vi "Playback.vi"() -> ()   [LabVIEW 2018]
doc: "This VI reads records of data from the logging table in the LabVIEW.mdb database. \n\nAll the records from the table are retrieved at one time using the DB Tools Select Data VI. This data is in the format of a two dimensional array of variants. This array is indexed and each of the values are converted back to their original data types."
uses:
  database example subvis/Fetching - State.ctl
  <vilib>/addons/database/Connection.llb/Conn ObjectReference.ctl
  <vilib>/addons/database/Connection.llb/DB Tools Open Connec (Path).vi
  <vilib>/addons/database/_DB Variant To Data/Database Variant To Data.xnode
  <vilib>/addons/database/NI_Database_API.lvlib
panel:
  out "record number":i32
  in  "Previous Record":bool
  in  "Next Record":bool
  in  "Stop":bool
  out "min temperature value":dbl format="%#.6g"
  out "max temperature value":dbl format="%#.6g"
  out "min pressure value":dbl format="%#.6g"
  out "max pressure value":dbl format="%#.6g"
  out "Core Temperature":dbl[](graph)
  out "Core Pressure":dbl[](graph)
  # "Overview: Demonstrates how to fetch the contents of an entire table from a database for playback.\nRequirements: Database Connectivity Toolkit\nInstructions:\n1. Make sure you have already run one of the \"Database Logging\" examples.\n2. Run this VI.\n3. Click the Previous Record and Next Record buttons to display individual records from the database.\n4. Click Stop to stop the VI."
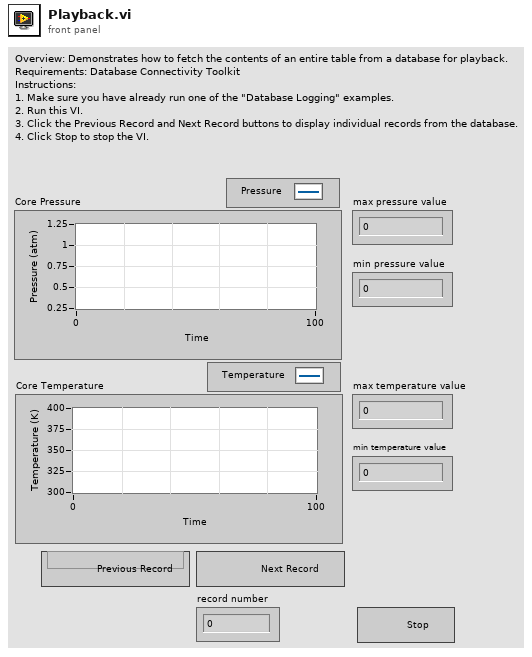
[diagram p1: front panel]
types:
  T1 = typedef "NI_Database_API.lvlib/Conn ObjectReference.ctl" = refnum<k1>
  T2 = typedef "Fetching - State.ctl" = enum16{"Initialize", "Wait for Event", "Prepare for Next", "Prepare for Previous", "Query Database", "Exit"}
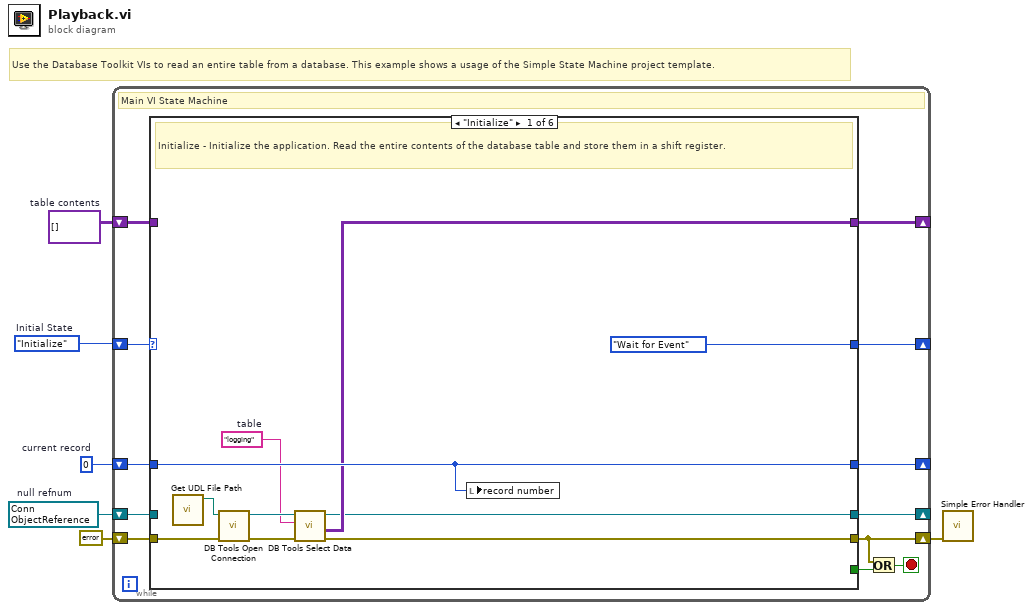
[diagram p0: block diagram]
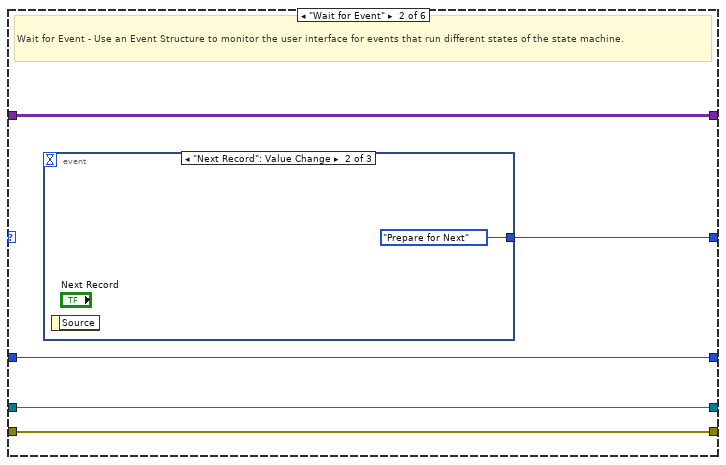
[diagram p2: hidden frame]
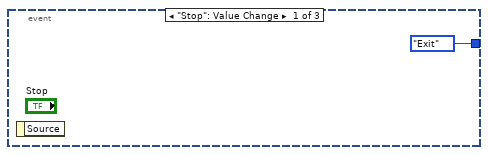
[diagram p3: hidden frame]
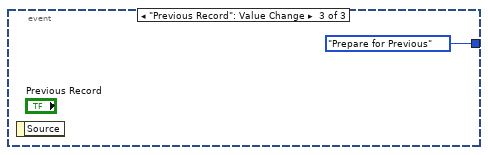
[diagram p4: hidden frame]
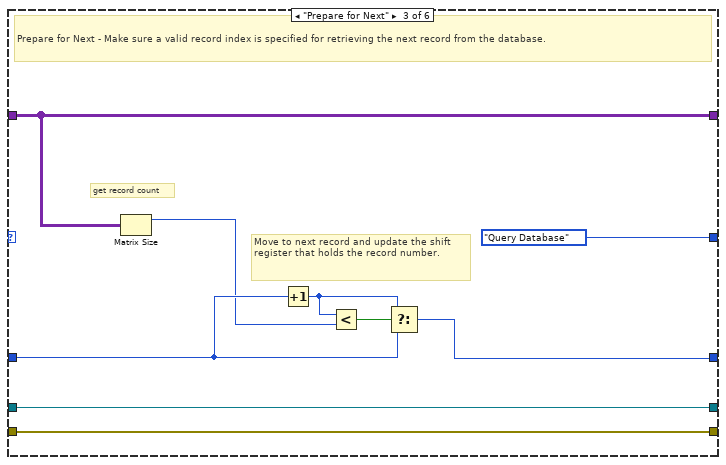
[diagram p5: hidden frame]
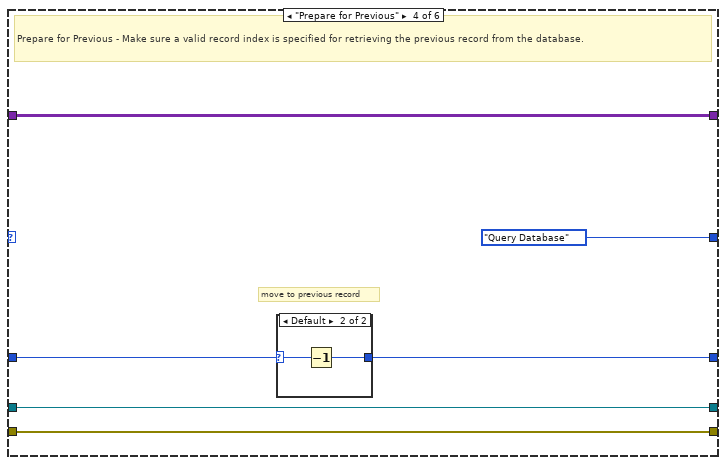
[diagram p6: hidden frame]
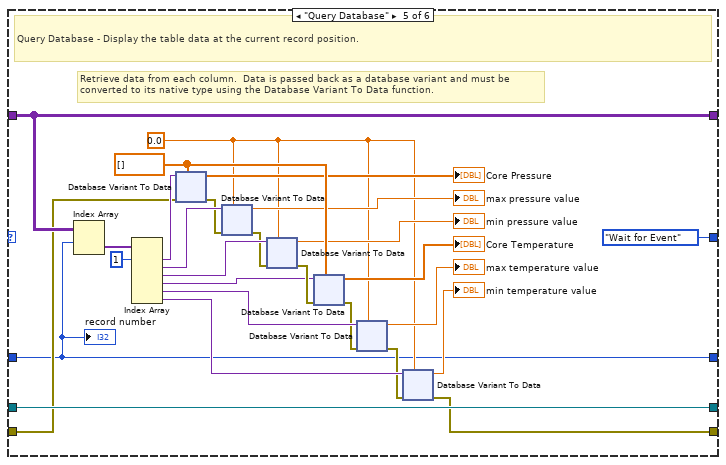
[diagram p8: hidden frame]
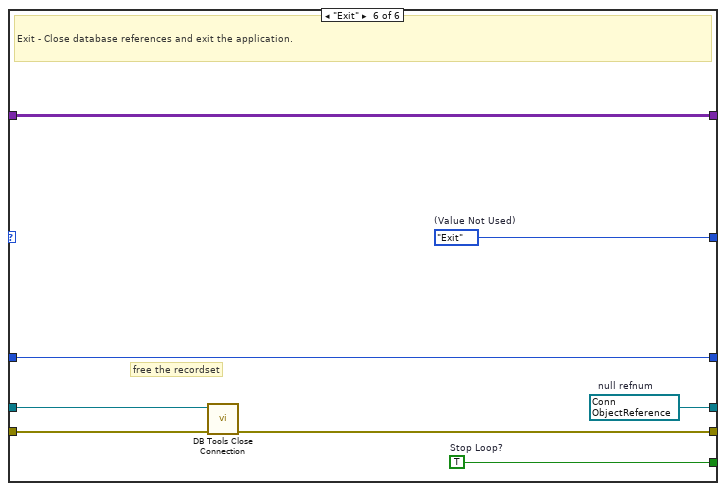
[diagram p9: hidden frame]
diagram:
  w1 = T1 refnum items=["Connection"]  # null refnum
  w2 = variant[][] []  # table contents
  w6 = 0  # current record
  w5 = Fetching_-_State."Initialize"  # Initial State
  # "Use the Database Toolkit VIs to read an entire table from a database. This example shows a usage of the Simple State Machine project template."
  n1 = while {
    shift-right: [w17] -> _
    shift-left: w5 -> [w18]
    shift-right: [w13] -> w3
    shift-left: errorcluster {"status"=FALSE, "code"=0, "source"=""} ("error constant") -> [w16]
    shift-right: [w12] -> _
    shift-left: w1 -> [w11]
    shift-right: [w9] -> _
    shift-left: w6 -> [w10]
    shift-right: [w8] -> _
    shift-left: w2 -> [w7]
    stop <- w14 stop-if-true
    # "Main VI State Machine"
    n2 = case shown="\"Initialize\"" w18 {
      tunnel: [Fetching_-_State."Wait for Event" ("(Value Not Used)") w33 Fetching_-_State."Query Database" ("(Value Not Used)") Fetching_-_State."Query Database" ("(Value Not Used)") Fetching_-_State."Wait for Event" ("(Value Not Used)") w287] -> w17
      tunnel: [_ _ _ _ _ w286] -> w15
      tunnel: w16 -> [w27 w31 w45 w51 w59 w285]
      tunnel: [w23 w31 w45 w51 w58 w284] -> w13
      tunnel: [w19 w32 w43 w49 w80 w281] -> w12
      tunnel: w11 -> [_ w32 w43 w49 w80 w282]
      tunnel: w10 -> [w25 w30 w39 w47 w56 w283]
      tunnel: [w25 w30 w40 w46 w56 w283] -> w9
      tunnel: [w20 w29 w38 w48 w61 w280] -> w8
      tunnel: w7 -> [_ w29 w38 w48 w61 w280]
      frame "Initialize" {
        w21 = "logging"  # table
        # "Initialize - Initialize the application. Read the entire contents of the database table and store them in a shift register."
        n3 = call "Get UDL File Path.vi"() -> ("UDL file path"=w28:path)  [unwired: 11 in]
        n4 = call-poly <vilib>:"DB Tools Open Connection.vi"("error in (no error)"=w27, "connection information"=w28) -> ("error out"=w24:errorcluster, "connection reference"=w22:T1)  [unwired: 6 in]
        n5 = call <vilib>:"DB Tools Select Data.vi"("error in (no error)"=w24, "table"=w21, "connection reference"=w22) -> ("error out"=w23:errorcluster, "data"=w20:variant[][], "connection reference out"=w19:T1)  [unwired: 3 in]
        n6 = local write "record number"(w25) -> ()
      }
      frame "Wait for Event" {
        # "Wait for Event - Use an Event Structure to monitor the user interface for events that run different states of the state machine."
        n7 = event shown="[1] \"Next Record\": Value Change" {
          selector: _ -> [_ _ _]
          dyn-events: _ -> [_ _ _]
          timeout: _ -> [_ _ _]
          tunnel: [Fetching_-_State."Exit" ("Next State") Fetching_-_State."Prepare for Next" ("Next State") Fetching_-_State."Prepare for Previous" ("Next State")] -> w33
          event "Stop": Value Change {
            n8 = event-data() -> ()  [unwired: 1 in, 1 out]
          }
          event "Next Record": Value Change {
            n9 = event-data() -> ()  [unwired: 1 in, 1 out]
          }
          event "Previous Record": Value Change {
            n10 = event-data() -> ()  [unwired: 1 in, 1 out]
          }
        }
      }
      frame "Prepare for Next" {
        # "get record count"
        # "Move to next record and update the shift register that holds the record number."
        # "Prepare for Next - Make sure a valid record index is specified for retrieving the next record from the database."
        n11 = Matrix Size(0:w38) -> (1:w37:i32)  [unwired: 1 out]
        n12 = Increment(x=w39) -> (x+1=w42:i32)
        n13 = Less?(x=w42, y=w37) -> (x < y?=w41:bool)
        n14 = Select(t=w42, s=w41, f=w39) -> (s? t:f=w40:i32)
      }
      frame "Prepare for Previous" {
        # "move to previous record"
        # "Prepare for Previous - Make sure a valid record index is specified for retrieving the previous record from the database."
        n15 = case shown="Default" w47 {
          selector: w47 -> [w52 w53]
          tunnel: [w52 w54] -> w46
          frame 0 {
          }
          frame Default {
            n16 = Decrement(x=w53) -> (x-1=w54:i32)
          }
        }
      }
      frame "Query Database" {
        w57 = 0.0
        w79 = dbl[] [] ("Array Constant")
        # "Retrieve data from each column.  Data is passed back as a database variant and must be converted to its native type using the Database Variant To Data function."
        # "Query Database - Display the table data at the current record position."
        n17 = Index Array(array=w61, index (row)=w56) -> (element=w62:variant[])  [unwired: 1 in]
        n18 = Index Array(array=w62, index #1=1) -> (element #1=w72:variant, element #2=w73:variant, element #3=w74:variant, element #4=w75:variant, element #5=w76:variant, element #6=w77:variant)  [unwired: 5 in]
        n19 = xnode "Database Variant To Data"("database variant"=w72, "error in (no error)"=w59, "type"=w79) -> ("data"=→"Core Pressure":dbl[], "error out"=w71:errorcluster)
        n20 = xnode "Database Variant To Data"("database variant"=w73, "error in (no error)"=w71, "type"=w57) -> ("data"=→"max pressure value":dbl, "error out"=w69:errorcluster)
        n21 = xnode "Database Variant To Data"("database variant"=w74, "error in (no error)"=w69, "type"=w57) -> ("data"=→"min pressure value":dbl, "error out"=w78:errorcluster)
        n22 = xnode "Database Variant To Data"("database variant"=w75, "error in (no error)"=w78, "type"=w79) -> ("data"=→"Core Temperature":dbl[], "error out"=w70:errorcluster)
        n23 = xnode "Database Variant To Data"("database variant"=w76, "error in (no error)"=w70, "type"=w57) -> ("data"=→"max temperature value":dbl, "error out"=w60:errorcluster)
        n24 = xnode "Database Variant To Data"("database variant"=w77, "error in (no error)"=w60, "type"=w57) -> ("data"=→"min temperature value":dbl, "error out"=w58:errorcluster)
        "record number" <- w56
      }
      frame "Exit" {
        w281 = T1 refnum items=["Connection"]  # null refnum
        w286 = TRUE  # Stop Loop?
        w287 = Fetching_-_State."Exit"  # (Value Not Used)
        # "free the recordset"
        # "Exit - Close database references and exit the application."
        n25 = call <vilib>:"DB Tools Close Connection.vi"("error in (no error)"=w285, "connection reference"=w282) -> ("error out"=w284:errorcluster)  [unwired: 5 in]
      }
    }
    n26 = Or(x=w13, y=w15) -> (x .or. y?=w14:bool)
  }
  n27 = call <vilib>:"Simple Error Handler.vi"("error in (no error)"=w3) -> ()  [unwired: 4 in, 5 out]
